vi "InverseKinematics.vi"(10 "X":dbl, 11 "Y":dbl) -> (2 "Q2":dbl, 3 "Q1":dbl)   [LabVIEW 2017]
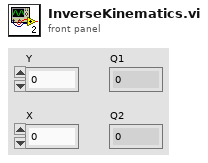
[diagram p1: front panel]
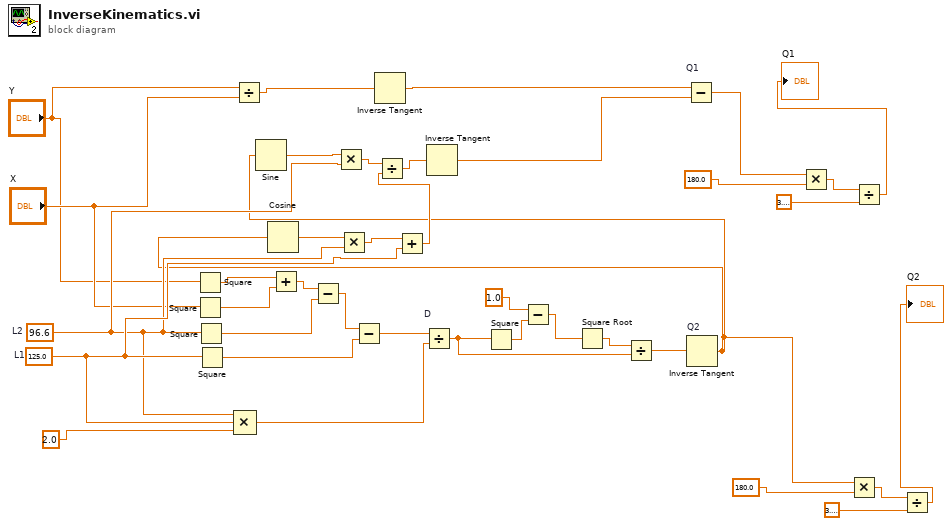
[diagram p0: block diagram]
diagram:
  w37 = 125.0  # L1
  w35 = 96.6  # L2
  n1 = Square(x="Y") -> (x^2=w13:dbl)
  n2 = Square(x="X") -> (x^2=w14:dbl)
  n3 = Square(x=w35) -> (x^2=w16:dbl)
  n4 = Square(x=w37) -> (x^2=w18:dbl)
  n5 = Divide(x="Y", y="X") -> (x/y=w28:dbl)
  n6 = Compound Arithmetic op=MULTIPLY(w35, w37, 2.0) -> (w21:dbl)
  n7 = Add(x=w13, y=w14) -> (x+y=w15:dbl)
  n8 = Subtract(x=w15, y=w16) -> (x-y=w17:dbl)
  n9 = Subtract(x=w17, y=w18) -> (x-y=w19:dbl)
  n10 = Inverse Tangent(1:w28) -> (0:w29:dbl)
  n11 = Divide "D"(x=w19, y=w21) -> (x/y=w26:dbl)
  n12 = Square(x=w26) -> (x^2=w25:dbl)
  n13 = Subtract(x=1.0, y=w25) -> (x-y=w27:dbl)
  n14 = Square Root(x=w27) -> (sqrt(x)=w23:dbl)
  n15 = Divide(x=w23, y=w26) -> (x/y=w22:dbl)
  n16 = Inverse Tangent "Q2"(1:w22) -> (0:w2:dbl)
  n17 = Sine(x=w2) -> (sin(x)=w31:dbl)
  n18 = Cosine(x=w2) -> (cos(x)=w34:dbl)
  n19 = Multiply(x=w31, y=w35) -> (x*y=w32:dbl)
  n20 = Multiply(x=w34, y=w35) -> (x*y=w36:dbl)
  n21 = Add(x=w36, y=w37) -> (x+y=w38:dbl)
  n22 = Divide(x=w32, y=w38) -> (x/y=w33:dbl)
  n23 = Inverse Tangent(1:w33) -> (0:w30:dbl)
  n24 = Subtract "Q1"(x=w29, y=w30) -> (x-y=w6:dbl)
  n25 = Multiply(x=w6, y=180.0) -> (x*y=w9:dbl)
  n26 = Multiply(x=w2, y=180.0) -> (x*y=w4:dbl)
  n27 = Divide(x=w9, y=3.141592653589793) -> (x/y=→"Q1":dbl)
  n28 = Divide(x=w4, y=3.141592653589793) -> (x/y=→"Q2":dbl)
